vi "PicoLogHRDL2.vi"(1 "stop":bool, 2 "Mains Frequency":i16(ring) items=["50 Hz", "60 Hz"], 3 "sampleInterval_ms":i32=1000, 4 "1":bool=TRUE) -> (0 "Waveform Graph":dynamicdata(graph))   [LabVIEW 2014]
uses:
  Instance           1 22Saved   HRDL_streaming .vi
  Instance           3 22Saved   HRDL_streaming .vi
  Instance           2 22Saved   HRDL_streaming .vi
  Instance           6 22Saved   HRDL_streaming .vi
  Instance           5 22Saved   HRDL_streaming .vi
  Instance           4 22Saved   HRDL_streaming .vi
  Instance          10 22Saved   HRDL_streaming .vi
  Instance           9 22Saved   HRDL_streaming .vi
  Instance           8 22Saved   HRDL_streaming .vi
  Instance           7 22Saved   HRDL_streaming .vi
  Instance          15 22Saved   HRDL_streaming .vi
  Instance          14 22Saved   HRDL_streaming .vi
  Instance          13 22Saved   HRDL_streaming .vi
  Instance          12 22Saved   HRDL_streaming .vi
  Instance          11 22Saved   HRDL_streaming .vi
  Instance          21 22Saved   HRDL_streaming .vi
  Instance          20 22Saved   HRDL_streaming .vi
  Instance          19 22Saved   HRDL_streaming .vi
  Instance          18 22Saved   HRDL_streaming .vi
  Instance          17 22Saved   HRDL_streaming .vi
  Instance          16 22Saved   HRDL_streaming .vi
  Instance          28 22Saved   HRDL_streaming .vi
  Instance          27 22Saved   HRDL_streaming .vi
  Instance          26 22Saved   HRDL_streaming .vi
  Instance          25 22Saved   HRDL_streaming .vi
  Instance          24 22Saved   HRDL_streaming .vi
  Instance          23 22Saved   HRDL_streaming .vi
  Instance          22 22Saved   HRDL_streaming .vi
  Instance          36 22Saved   HRDL_streaming .vi
  Instance          35 22Saved   HRDL_streaming .vi
  Instance          34 22Saved   HRDL_streaming .vi
  Instance          33 22Saved   HRDL_streaming .vi
  Instance          32 22Saved   HRDL_streaming .vi
  Instance          31 22Saved   HRDL_streaming .vi
  Instance          30 22Saved   HRDL_streaming .vi
  Instance          29 22Saved   HRDL_streaming .vi
  Instance          45 22Saved   HRDL_streaming .vi
  Instance          44 22Saved   HRDL_streaming .vi
  Instance          43 22Saved   HRDL_streaming .vi
  Instance          42 22Saved   HRDL_streaming .vi
  Instance          41 22Saved   HRDL_streaming .vi
  Instance          40 22Saved   HRDL_streaming .vi
  Instance          39 22Saved   HRDL_streaming .vi
  Instance          38 22Saved   HRDL_streaming .vi
  Instance          37 22Saved   HRDL_streaming .vi
  Instance          55 22Saved   HRDL_streaming .vi
  Instance          54 22Saved   HRDL_streaming .vi
  Instance          53 22Saved   HRDL_streaming .vi
  Instance          52 22Saved   HRDL_streaming .vi
  Instance          51 22Saved   HRDL_streaming .vi
  Instance          50 22Saved   HRDL_streaming .vi
  Instance          49 22Saved   HRDL_streaming .vi
  Instance          48 22Saved   HRDL_streaming .vi
  Instance          47 22Saved   HRDL_streaming .vi
  Instance          46 22Saved   HRDL_streaming .vi
  Instance          66 22Saved   HRDL_streaming .vi
  Instance          65 22Saved   HRDL_streaming .vi
  Instance          64 22Saved   HRDL_streaming .vi
  Instance          63 22Saved   HRDL_streaming .vi
  Instance          62 22Saved   HRDL_streaming .vi
  Instance          61 22Saved   HRDL_streaming .vi
  Instance          60 22Saved   HRDL_streaming .vi
  Instance          59 22Saved   HRDL_streaming .vi
  Instance          58 22Saved   HRDL_streaming .vi
  Instance          57 22Saved   HRDL_streaming .vi
  Instance          56 22Saved   HRDL_streaming .vi
  Instance          78 22Saved   HRDL_streaming .vi
  Instance          77 22Saved   HRDL_streaming .vi
  Instance          76 22Saved   HRDL_streaming .vi
  Instance          75 22Saved   HRDL_streaming .vi
  Instance          74 22Saved   HRDL_streaming .vi
  Instance          73 22Saved   HRDL_streaming .vi
  Instance          72 22Saved   HRDL_streaming .vi
  Instance          71 22Saved   HRDL_streaming .vi
  Instance          70 22Saved   HRDL_streaming .vi
  Instance          69 22Saved   HRDL_streaming .vi
  Instance          68 22Saved   HRDL_streaming .vi
  Instance          67 22Saved   HRDL_streaming .vi
  Instance          91 22Saved   HRDL_streaming .vi
  Instance          90 22Saved   HRDL_streaming .vi
  Instance          89 22Saved   HRDL_streaming .vi
  Instance          88 22Saved   HRDL_streaming .vi
  Instance          87 22Saved   HRDL_streaming .vi
  Instance          86 22Saved   HRDL_streaming .vi
  Instance          85 22Saved   HRDL_streaming .vi
  Instance          84 22Saved   HRDL_streaming .vi
  Instance          83 22Saved   HRDL_streaming .vi
  Instance          82 22Saved   HRDL_streaming .vi
  Instance          81 22Saved   HRDL_streaming .vi
  Instance          80 22Saved   HRDL_streaming .vi
  Instance          79 22Saved   HRDL_streaming .vi
  Instance         105 22Saved   HRDL_streaming .vi
  Instance         104 22Saved   HRDL_streaming .vi
  Instance         103 22Saved   HRDL_streaming .vi
  Instance         102 22Saved   HRDL_streaming .vi
  Instance         101 22Saved   HRDL_streaming .vi
  Instance         100 22Saved   HRDL_streaming .vi
  Instance          99 22Saved   HRDL_streaming .vi
  Instance          98 22Saved   HRDL_streaming .vi
  Instance          97 22Saved   HRDL_streaming .vi
  Instance          96 22Saved   HRDL_streaming .vi
  Instance          95 22Saved   HRDL_streaming .vi
  Instance          94 22Saved   HRDL_streaming .vi
  Instance          93 22Saved   HRDL_streaming .vi
  Instance          92 22Saved   HRDL_streaming .vi
  Instance         120 22Saved   HRDL_streaming .vi
  Instance         119 22Saved   HRDL_streaming .vi
  Instance         118 22Saved   HRDL_streaming .vi
  Instance         117 22Saved   HRDL_streaming .vi
  Instance         116 22Saved   HRDL_streaming .vi
  Instance         115 22Saved   HRDL_streaming .vi
  Instance         114 22Saved   HRDL_streaming .vi
  Instance         113 22Saved   HRDL_streaming .vi
  Instance         112 22Saved   HRDL_streaming .vi
  Instance         111 22Saved   HRDL_streaming .vi
  Instance         110 22Saved   HRDL_streaming .vi
  Instance         109 22Saved   HRDL_streaming .vi
  Instance         108 22Saved   HRDL_streaming .vi
  Instance         107 22Saved   HRDL_streaming .vi
  Instance         106 22Saved   HRDL_streaming .vi
  Instance         136 22Saved   HRDL_streaming .vi
  Instance         135 22Saved   HRDL_streaming .vi
  Instance         134 22Saved   HRDL_streaming .vi
  Instance         133 22Saved   HRDL_streaming .vi
  Instance         132 22Saved   HRDL_streaming .vi
  Instance         131 22Saved   HRDL_streaming .vi
  Instance         130 22Saved   HRDL_streaming .vi
  Instance         129 22Saved   HRDL_streaming .vi
  Instance         128 22Saved   HRDL_streaming .vi
  Instance         127 22Saved   HRDL_streaming .vi
  Instance         126 22Saved   HRDL_streaming .vi
  Instance         125 22Saved   HRDL_streaming .vi
  Instance         124 22Saved   HRDL_streaming .vi
  Instance         123 22Saved   HRDL_streaming .vi
  Instance         122 22Saved   HRDL_streaming .vi
  Instance         121 22Saved   HRDL_streaming .vi
  Instance         137 22Saved   HRDL_streaming .vi
  Instance         138 22Saved   HRDL_streaming .vi
  picohrdl.dll
panel:
  out "Unit Info":T1
  in  "conversionTime":i16(ring) items=["60 ms", "100 ms", "180 ms", "340 ms", "660 ms"]
  out "noOfChannels":i16=2
  in  "16":bool
  in  "15":bool
  in  "14":bool
  in  "13":bool
  in  "12":bool
  in  "11":bool
  in  "10":bool
  in  "9":bool
  in  "8":bool
  in  "7":bool
  in  "6":bool
  in  "5":bool
  in  "4":bool
  in  "3":bool
  in  "2":bool=TRUE
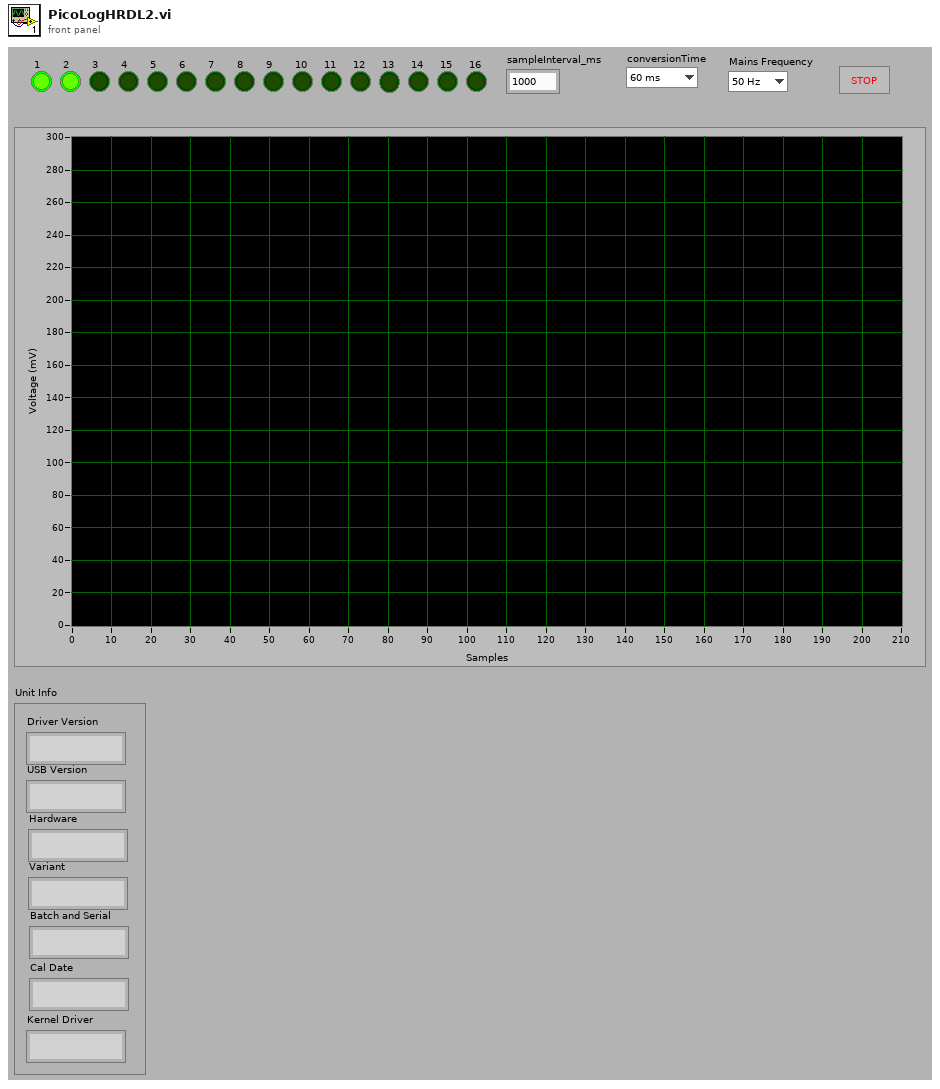
[diagram p1: front panel]
types:
  T1 = cluster{"Driver Version":string, "USB Version":string, "Hardware":string, "Variant":string, "Batch and Serial":string, "Cal Date":string, "Kernel Driver":string}
  T2 = cluster{"[0]":string, "[1]":string, "[2]":string, "[3]":string, "[4]":string, "[5]":string, "[6]":string}
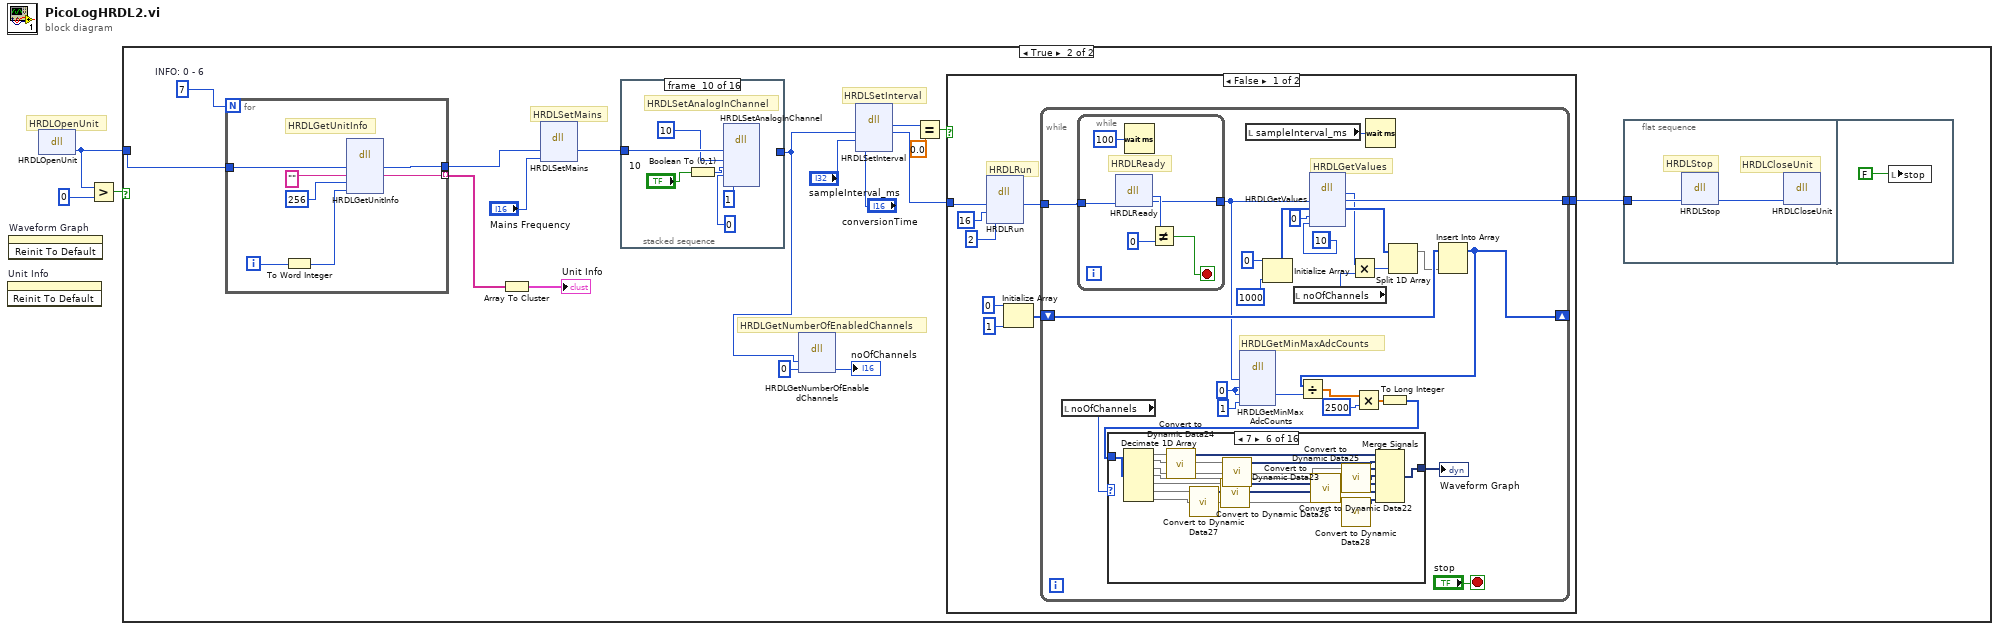
[diagram p0: block diagram]
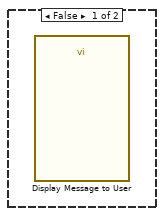
[diagram p2: hidden frame]
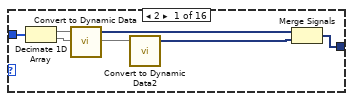
[diagram p3: hidden frame]
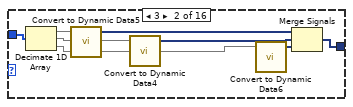
[diagram p4: hidden frame]
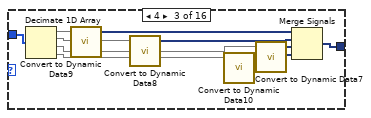
[diagram p5: hidden frame]
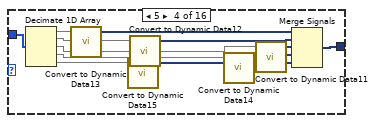
[diagram p6: hidden frame]
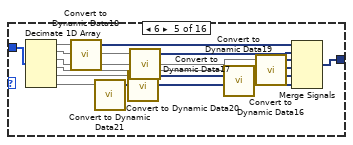
[diagram p7: hidden frame]
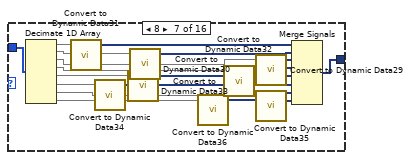
[diagram p8: hidden frame]
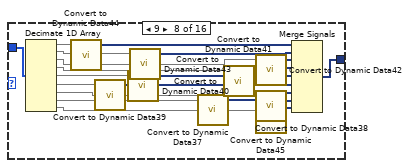
[diagram p9: hidden frame]
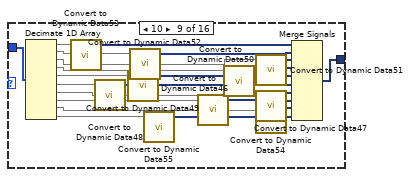
[diagram p10: hidden frame]
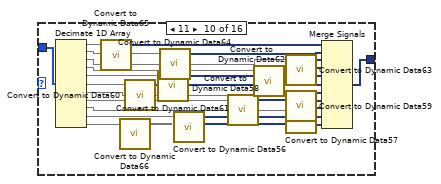
[diagram p11: hidden frame]
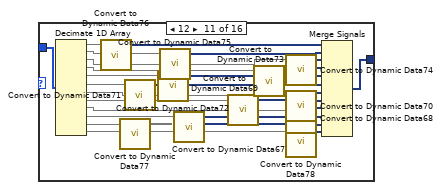
[diagram p12: hidden frame]
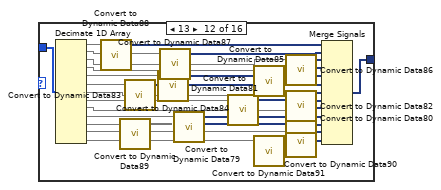
[diagram p13: hidden frame]
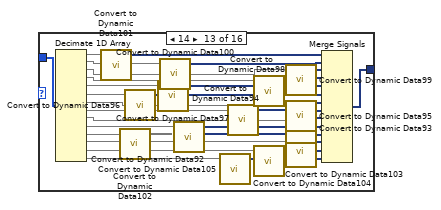
[diagram p14: hidden frame]
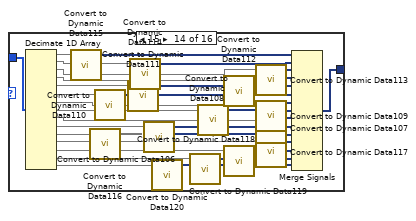
[diagram p15: hidden frame]
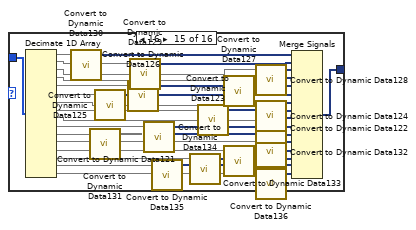
[diagram p16: hidden frame]
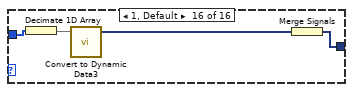
[diagram p17: hidden frame]
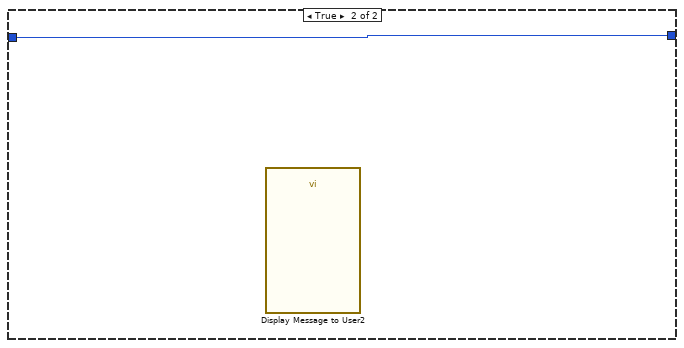
[diagram p18: hidden frame]
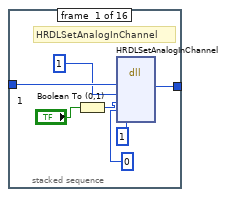
[diagram p19: hidden frame]
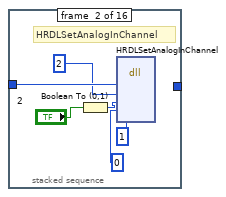
[diagram p20: hidden frame]
diagram:
  # "HRDLOpenUnit"
  n1 = invoke on="Unit Info" class="Clust (strict)" method="Reinit To Default"() -> ()  [unwired: 3 in, 3 out]
  n2 = invoke on="Waveform Graph" class="WFGraph (strict)" method="Reinit To Default"() -> ()  [unwired: 3 in, 3 out]
  n3 = dll-call lib="picohrdl.dll" fn="HRDLOpenUnit"() -> ("handle"=w1:i16)  [unwired: 3 in, 2 out]
  n4 = Greater?(x=w1, y=i16 0) -> (0:w3:bool)
  n5 = case shown="True" w3 {
    tunnel: w1 -> [_ w6]
    frame False {
      n6 = call "Display Message to User"() -> ()  [unwired: 10 in, 2 out]
    }
    frame True {
      w8 = 7  # INFO: 0 - 6
      # "HRDLGetNumberOfEnabledChannels"
      # "HRDLSetInterval"
      # "HRDLSetMains"
      n7 = for {
        N: w8 -> [_]
        tunnel: w6 -> [w27]
        tunnel: [w24] -> w5 mode=indexing
        tunnel: [w22] -> w7
        i -> [w23]
        # "HRDLGetUnitInfo"
        n8 = To Word Integer(number=w23) -> (16bit integer=w21:i16)
        n9 = dll-call lib="picohrdl.dll" fn="HRDLGetUnitInfo"("handle"=w27, "unitInfo"="", "stringLength"=i16 256, "info"=w21) -> ("handle"=w22:i16, "unitInfo"=w24:string)  [unwired: 6 in, 2 out]
      }
      n10 = Array To Cluster(array=w5) -> (cluster=→"Unit Info":T2)
      n11 = dll-call lib="PicoHRDL.dll" fn="HRDLSetMains"("handle"=w7, "sixtyHertz"="Mains Frequency") -> ("handle"=w11:i16)  [unwired: 5 in, 2 out]
      n12 = stacked-sequence {
        tunnel: w11 -> [w379 w385 w391 w397 w403 w409 w415 w421 w427 w433 w439 w445 w451 w457 w463 w469]
        tunnel: [w378 _ _ _ _ _ _ _ _ _ _ _ _ _ _ _] -> w9
        frame #0 {
          # "HRDLSetAnalogInChannel"
          n13 = Boolean To (0,1)(Boolean="1") -> (0, 1=w373:i16)
          n14 = dll-call lib="PicoHRDL.dll" fn="HRDLSetAnalogInChannel"("handle"=w379, "channel"=i16 1, "enabled"=w373, "range"=i16 0 ("range 1"), "singleEnded"=i16 1) -> ("handle"=w378:i16)  [unwired: 8 in, 2 out]
        }
        frame #1 {
          # "HRDLSetAnalogInChannel"
          n15 = Boolean To (0,1)(Boolean="2") -> (0, 1=w381:i16)
          n16 = dll-call lib="PicoHRDL.dll" fn="HRDLSetAnalogInChannel"("handle"=w385, "channel"=i16 2, "enabled"=w381, "range"=i16 0 ("range 2"), "singleEnded"=i16 1) -> ()  [unwired: 9 in, 2 out]
        }
        frame #2 {
          # "HRDLSetAnalogInChannel"
          n17 = Boolean To (0,1)(Boolean="3") -> (0, 1=w387:i16)
          n18 = dll-call lib="PicoHRDL.dll" fn="HRDLSetAnalogInChannel"("handle"=w391, "channel"=i16 3, "enabled"=w387, "range"=i16 0 ("range 3"), "singleEnded"=i16 1) -> ()  [unwired: 9 in, 2 out]
        }
        frame #3 {
          # "HRDLSetAnalogInChannel"
          n19 = Boolean To (0,1)(Boolean="4") -> (0, 1=w393:i16)
          n20 = dll-call lib="PicoHRDL.dll" fn="HRDLSetAnalogInChannel"("handle"=w397, "channel"=i16 4, "enabled"=w393, "range"=i16 0 ("range 4"), "singleEnded"=i16 1) -> ()  [unwired: 9 in, 2 out]
        }
        frame #4 {
          # "HRDLSetAnalogInChannel"
          n21 = Boolean To (0,1)(Boolean="5") -> (0, 1=w399:i16)
          n22 = dll-call lib="PicoHRDL.dll" fn="HRDLSetAnalogInChannel"("handle"=w403, "channel"=i16 5, "enabled"=w399, "range"=i16 0 ("range 5"), "singleEnded"=i16 1) -> ()  [unwired: 9 in, 2 out]
        }
        frame #5 {
          # "HRDLSetAnalogInChannel"
          n23 = Boolean To (0,1)(Boolean="6") -> (0, 1=w405:i16)
          n24 = dll-call lib="PicoHRDL.dll" fn="HRDLSetAnalogInChannel"("handle"=w409, "channel"=i16 6, "enabled"=w405, "range"=i16 0 ("range 6"), "singleEnded"=i16 1) -> ()  [unwired: 9 in, 2 out]
        }
        frame #6 {
          # "HRDLSetAnalogInChannel"
          n25 = Boolean To (0,1)(Boolean="7") -> (0, 1=w411:i16)
          n26 = dll-call lib="PicoHRDL.dll" fn="HRDLSetAnalogInChannel"("handle"=w415, "channel"=i16 7, "enabled"=w411, "range"=i16 0 ("range 7"), "singleEnded"=i16 1) -> ()  [unwired: 9 in, 2 out]
        }
        frame #7 {
          # "HRDLSetAnalogInChannel"
          n27 = Boolean To (0,1)(Boolean="8") -> (0, 1=w417:i16)
          n28 = dll-call lib="PicoHRDL.dll" fn="HRDLSetAnalogInChannel"("handle"=w421, "channel"=i16 8, "enabled"=w417, "range"=i16 0 ("range 8"), "singleEnded"=i16 1) -> ()  [unwired: 9 in, 2 out]
        }
        frame #8 {
          # "HRDLSetAnalogInChannel"
          n29 = Boolean To (0,1)(Boolean="9") -> (0, 1=w423:i16)
          n30 = dll-call lib="PicoHRDL.dll" fn="HRDLSetAnalogInChannel"("handle"=w427, "channel"=i16 9, "enabled"=w423, "range"=i16 0 ("range 9"), "singleEnded"=i16 1) -> ()  [unwired: 9 in, 2 out]
        }
        frame #9 {
          # "HRDLSetAnalogInChannel"
          n31 = Boolean To (0,1)(Boolean="10") -> (0, 1=w429:i16)
          n32 = dll-call lib="PicoHRDL.dll" fn="HRDLSetAnalogInChannel"("handle"=w433, "channel"=i16 10, "enabled"=w429, "range"=i16 0 ("range 10"), "singleEnded"=i16 1) -> ()  [unwired: 9 in, 2 out]
        }
        frame #10 {
          # "HRDLSetAnalogInChannel"
          n33 = Boolean To (0,1)(Boolean="11") -> (0, 1=w435:i16)
          n34 = dll-call lib="PicoHRDL.dll" fn="HRDLSetAnalogInChannel"("handle"=w439, "channel"=i16 11, "enabled"=w435, "range"=i16 0 ("range 11"), "singleEnded"=i16 1) -> ()  [unwired: 9 in, 2 out]
        }
        frame #11 {
          # "HRDLSetAnalogInChannel"
          n35 = Boolean To (0,1)(Boolean="12") -> (0, 1=w441:i16)
          n36 = dll-call lib="PicoHRDL.dll" fn="HRDLSetAnalogInChannel"("handle"=w445, "channel"=i16 12, "enabled"=w441, "range"=i16 0 ("range 12"), "singleEnded"=i16 1) -> ()  [unwired: 9 in, 2 out]
        }
        frame #12 {
          # "HRDLSetAnalogInChannel"
          n37 = Boolean To (0,1)(Boolean="13") -> (0, 1=w447:i16)
          n38 = dll-call lib="PicoHRDL.dll" fn="HRDLSetAnalogInChannel"("handle"=w451, "channel"=i16 13, "enabled"=w447, "range"=i16 0 ("range 13"), "singleEnded"=i16 1) -> ()  [unwired: 9 in, 2 out]
        }
        frame #13 {
          # "HRDLSetAnalogInChannel"
          n39 = Boolean To (0,1)(Boolean="14") -> (0, 1=w453:i16)
          n40 = dll-call lib="PicoHRDL.dll" fn="HRDLSetAnalogInChannel"("handle"=w457, "channel"=i16 14, "enabled"=w453, "range"=i16 0 ("range 14"), "singleEnded"=i16 1) -> ()  [unwired: 9 in, 2 out]
        }
        frame #14 {
          # "HRDLSetAnalogInChannel"
          n41 = Boolean To (0,1)(Boolean="15") -> (0, 1=w459:i16)
          n42 = dll-call lib="PicoHRDL.dll" fn="HRDLSetAnalogInChannel"("handle"=w463, "channel"=i16 15, "enabled"=w459, "range"=i16 0 ("range 15"), "singleEnded"=i16 1) -> ()  [unwired: 9 in, 2 out]
        }
        frame #15 {
          # "HRDLSetAnalogInChannel"
          n43 = Boolean To (0,1)(Boolean="16") -> (0, 1=w465:i16)
          n44 = dll-call lib="PicoHRDL.dll" fn="HRDLSetAnalogInChannel"("handle"=w469, "channel"=i16 16, "enabled"=w465, "range"=i16 0 ("range 16"), "singleEnded"=i16 1) -> ()  [unwired: 9 in, 2 out]
        }
      }
      n45 = dll-call lib="PicoHRDL.dll" fn="HRDLGetNumberOfEnabledChannels"("handle"=w9, "nEnabledChannels"=i16 0) -> ("nEnabledChannels"=→"noOfChannels":i16)  [unwired: 5 in, 2 out]
      n46 = dll-call lib="PicoHRDL.dll" fn="HRDLSetInterval"("handle"=w9, "sampleInterval_ms"="sampleInterval_ms", "conversionTime"="conversionTime") -> ("return type"=w15:i16, "handle"=w14:i16)  [unwired: 5 in, 2 out]
      n47 = Equal?(x=w15, y=0.0) -> (x = y?=w13:bool)
      n48 = case shown="False" w13 {
        tunnel: [w32 w372] -> w20
        tunnel: w14 -> [w28 w372]
        frame False {
          # "HRDLRun"
          n49 = dll-call lib="PicoHRDL.dll" fn="HRDLRun"("handle"=w28, "nValues"=16, "method"=i16 2) -> ("handle"=w33:i16)  [unwired: 6 in, 2 out]
          n50 = Initialize Array(0 ("element"), 1 ("dimension size")) -> (w29:i32[])
          n51 = while {
            tunnel: w33 -> [w61]
            tunnel: [w55] -> w32
            shift-right: [w48] -> _
            shift-left: w29 -> [w49]
            stop <- "stop" stop-if-true
            w53 = 0 ("maxAdc")
            (unwired) 10 ("noOfValues")
            # "HRDLGetMinMaxAdcCounts"
            # "HRDLGetValues"
            n52 = local read "noOfChannels"() -> (w42:i16)
            n53 = while {
              tunnel: w61 -> [w368]
              tunnel: [w367] -> w38
              stop <- w369 stop-if-true
              # "HRDLReady"
              n54 = dll-call lib="PicoHRDL.dll" fn="HRDLReady"("handle"=w368) -> ("ready"=w371:i16, "handle"=w367:i16)  [unwired: 3 in, 2 out]
              n55 = Wait (ms)(milliseconds to wait=u32 100) -> ()  [unwired: 1 out]
              n56 = Not Equal?(x=w371, y=i16 0) -> (x != y?=w369:bool)
            }
            n57 = dll-call lib="PicoHRDL.dll" fn="HRDLGetMinMaxAdcCounts"("handle"=w38, "minAdc"=w53, "maxAdc"=w53, "channel"=i16 1) -> ("maxAdc"=w39:i32)  [unwired: 7 in, 2 out]
            n58 = local read "sampleInterval_ms"() -> (w36:i32)
            n59 = Initialize Array(0 ("element"), 1000 ("dimension size")) -> (w60:i32[])
            n60 = local read "noOfChannels"() -> (w46:i16)
            n61 = dll-call lib="PicoHRDL.dll" fn="HRDLGetValues"("handle"=w38, "values"=w60, "overflow"=i16 0, "noOfValues"=10) -> ("noValuesPerChan"=w44:i32, "handle"=w55:i16, "values"=w47:i32[])  [unwired: 5 in, 2 out]
            n62 = Multiply(x=w44, y=w46) -> (x*y=w45:i32)
            n63 = Wait (ms)(milliseconds to wait=w36) -> ()  [unwired: 1 out]
            n64 = Split 1D Array(array=w47, index=w45) -> (first subarray=w43:i32[])  [unwired: 1 out]
            n65 = Insert Into Array(array=w49, new element=w43) -> (w48:i32[])  [unwired: 1 in]
            n66 = Divide(x=w48, y=w39) -> (x/y=w52:dbl[])
            n67 = Multiply(x=w52, y=2500 ("noOfValues")) -> (x*y=w51:dbl[])
            n68 = To Long Integer(number=w51) -> (32bit integer=w40:i32[])
            n69 = case shown="7" w42 {
              tunnel: [w63 w71 w81 w93 w107 w123 w141 w161 w183 w207 w233 w261 w291 w323 w357 w363] -> w41
              tunnel: w40 -> [w62 w70 w80 w92 w106 w122 w140 w160 w182 w206 w232 w260 w290 w322 w356 w362]
              frame 2 {
                n70 = Decimate 1D Array(w62) -> (w64:i32[], w66:i32[])
                n71 = call "Convert to Dynamic Data"("Array"=w64) -> ("Dynamic Data Type"=w65:dynamicdata)  [unwired: 3 in]
                n72 = call "Convert to Dynamic Data2"("Array"=w66) -> ("Dynamic Data Type"=w67:dynamicdata)  [unwired: 3 in]
                n73 = Merge Signals(w65, w67) -> (w63:dynamicdata)
              }
              frame 3 {
                n74 = Decimate 1D Array(w70) -> (w72:i32[], w74:i32[], w69:i32[])
                n75 = call "Convert to Dynamic Data5"("Array"=w72) -> ("Dynamic Data Type"=w73:dynamicdata)  [unwired: 3 in]
                n76 = call "Convert to Dynamic Data4"("Array"=w74) -> ("Dynamic Data Type"=w75:dynamicdata)  [unwired: 3 in]
                n77 = call "Convert to Dynamic Data6"("Array"=w69) -> ("Dynamic Data Type"=w68:dynamicdata)  [unwired: 3 in]
                n78 = Merge Signals(w73, w75, w68) -> (w71:dynamicdata)
              }
              frame 4 {
                n79 = Decimate 1D Array(w80) -> (w82:i32[], w84:i32[], w79:i32[], w77:i32[])
                n80 = call "Convert to Dynamic Data9"("Array"=w82) -> ("Dynamic Data Type"=w83:dynamicdata)  [unwired: 3 in]
                n81 = call "Convert to Dynamic Data8"("Array"=w84) -> ("Dynamic Data Type"=w85:dynamicdata)  [unwired: 3 in]
                n82 = call "Convert to Dynamic Data10"("Array"=w77) -> ("Dynamic Data Type"=w76:dynamicdata)  [unwired: 3 in]
                n83 = call "Convert to Dynamic Data7"("Array"=w79) -> ("Dynamic Data Type"=w78:dynamicdata)  [unwired: 3 in]
                n84 = Merge Signals(w83, w85, w78, w76) -> (w81:dynamicdata)
              }
              frame 5 {
                n85 = Decimate 1D Array(w92) -> (w94:i32[], w96:i32[], w91:i32[], w89:i32[], w87:i32[])
                n86 = call "Convert to Dynamic Data13"("Array"=w94) -> ("Dynamic Data Type"=w95:dynamicdata)  [unwired: 3 in]
                n87 = call "Convert to Dynamic Data15"("Array"=w87) -> ("Dynamic Data Type"=w86:dynamicdata)  [unwired: 3 in]
                n88 = call "Convert to Dynamic Data12"("Array"=w96) -> ("Dynamic Data Type"=w97:dynamicdata)  [unwired: 3 in]
                n89 = call "Convert to Dynamic Data14"("Array"=w89) -> ("Dynamic Data Type"=w88:dynamicdata)  [unwired: 3 in]
                n90 = call "Convert to Dynamic Data11"("Array"=w91) -> ("Dynamic Data Type"=w90:dynamicdata)  [unwired: 3 in]
                n91 = Merge Signals(w95, w97, w90, w88, w86) -> (w93:dynamicdata)
              }
              frame 6 {
                n92 = Decimate 1D Array(w106) -> (w108:i32[], w110:i32[], w105:i32[], w103:i32[], w101:i32[], w99:i32[])
                n93 = call "Convert to Dynamic Data18"("Array"=w108) -> ("Dynamic Data Type"=w109:dynamicdata)  [unwired: 3 in]
                n94 = call "Convert to Dynamic Data21"("Array"=w99) -> ("Dynamic Data Type"=w98:dynamicdata)  [unwired: 3 in]
                n95 = call "Convert to Dynamic Data20"("Array"=w101) -> ("Dynamic Data Type"=w100:dynamicdata)  [unwired: 3 in]
                n96 = call "Convert to Dynamic Data17"("Array"=w110) -> ("Dynamic Data Type"=w111:dynamicdata)  [unwired: 3 in]
                n97 = call "Convert to Dynamic Data19"("Array"=w103) -> ("Dynamic Data Type"=w102:dynamicdata)  [unwired: 3 in]
                n98 = call "Convert to Dynamic Data16"("Array"=w105) -> ("Dynamic Data Type"=w104:dynamicdata)  [unwired: 3 in]
                n99 = Merge Signals(w109, w111, w104, w102, w100, w98) -> (w107:dynamicdata)
              }
              frame 7 {
                n100 = Decimate 1D Array(w122) -> (w124:i32[], w126:i32[], w121:i32[], w119:i32[], w117:i32[], w115:i32[], w113:i32[])
                n101 = call "Convert to Dynamic Data24"("Array"=w124) -> ("Dynamic Data Type"=w125:dynamicdata)  [unwired: 3 in]
                n102 = call "Convert to Dynamic Data27"("Array"=w115) -> ("Dynamic Data Type"=w114:dynamicdata)  [unwired: 3 in]
                n103 = call "Convert to Dynamic Data26"("Array"=w117) -> ("Dynamic Data Type"=w116:dynamicdata)  [unwired: 3 in]
                n104 = call "Convert to Dynamic Data23"("Array"=w126) -> ("Dynamic Data Type"=w127:dynamicdata)  [unwired: 3 in]
                n105 = call "Convert to Dynamic Data25"("Array"=w119) -> ("Dynamic Data Type"=w118:dynamicdata)  [unwired: 3 in]
                n106 = call "Convert to Dynamic Data22"("Array"=w121) -> ("Dynamic Data Type"=w120:dynamicdata)  [unwired: 3 in]
                n107 = call "Convert to Dynamic Data28"("Array"=w113) -> ("Dynamic Data Type"=w112:dynamicdata)  [unwired: 3 in]
                n108 = Merge Signals(w125, w127, w120, w118, w116, w114, w112) -> (w123:dynamicdata)
              }
              frame 8 {
                n109 = Decimate 1D Array(w140) -> (w142:i32[], w144:i32[], w139:i32[], w137:i32[], w135:i32[], w133:i32[], w131:i32[], w129:i32[])
                n110 = call "Convert to Dynamic Data31"("Array"=w142) -> ("Dynamic Data Type"=w143:dynamicdata)  [unwired: 3 in]
                n111 = call "Convert to Dynamic Data34"("Array"=w133) -> ("Dynamic Data Type"=w132:dynamicdata)  [unwired: 3 in]
                n112 = call "Convert to Dynamic Data33"("Array"=w135) -> ("Dynamic Data Type"=w134:dynamicdata)  [unwired: 3 in]
                n113 = call "Convert to Dynamic Data30"("Array"=w144) -> ("Dynamic Data Type"=w145:dynamicdata)  [unwired: 3 in]
                n114 = call "Convert to Dynamic Data36"("Array"=w129) -> ("Dynamic Data Type"=w128:dynamicdata)  [unwired: 3 in]
                n115 = call "Convert to Dynamic Data32"("Array"=w137) -> ("Dynamic Data Type"=w136:dynamicdata)  [unwired: 3 in]
                n116 = call "Convert to Dynamic Data29"("Array"=w139) -> ("Dynamic Data Type"=w138:dynamicdata)  [unwired: 3 in]
                n117 = call "Convert to Dynamic Data35"("Array"=w131) -> ("Dynamic Data Type"=w130:dynamicdata)  [unwired: 3 in]
                n118 = Merge Signals(w143, w145, w138, w136, w134, w132, w130, w128) -> (w141:dynamicdata)
              }
              frame 9 {
                n119 = Decimate 1D Array(w160) -> (w162:i32[], w164:i32[], w159:i32[], w157:i32[], w155:i32[], w153:i32[], w151:i32[], w149:i32[], w147:i32[])
                n120 = call "Convert to Dynamic Data44"("Array"=w162) -> ("Dynamic Data Type"=w163:dynamicdata)  [unwired: 3 in]
                n121 = call "Convert to Dynamic Data39"("Array"=w153) -> ("Dynamic Data Type"=w152:dynamicdata)  [unwired: 3 in]
                n122 = call "Convert to Dynamic Data40"("Array"=w155) -> ("Dynamic Data Type"=w154:dynamicdata)  [unwired: 3 in]
                n123 = call "Convert to Dynamic Data43"("Array"=w164) -> ("Dynamic Data Type"=w165:dynamicdata)  [unwired: 3 in]
                n124 = call "Convert to Dynamic Data37"("Array"=w149) -> ("Dynamic Data Type"=w148:dynamicdata)  [unwired: 3 in]
                n125 = call "Convert to Dynamic Data41"("Array"=w157) -> ("Dynamic Data Type"=w156:dynamicdata)  [unwired: 3 in]
                n126 = call "Convert to Dynamic Data42"("Array"=w159) -> ("Dynamic Data Type"=w158:dynamicdata)  [unwired: 3 in]
                n127 = call "Convert to Dynamic Data38"("Array"=w151) -> ("Dynamic Data Type"=w150:dynamicdata)  [unwired: 3 in]
                n128 = call "Convert to Dynamic Data45"("Array"=w147) -> ("Dynamic Data Type"=w146:dynamicdata)  [unwired: 3 in]
                n129 = Merge Signals(w163, w165, w158, w156, w154, w152, w150, w148, w146) -> (w161:dynamicdata)
              }
              frame 10 {
                n130 = Decimate 1D Array(w182) -> (w184:i32[], w186:i32[], w181:i32[], w179:i32[], w177:i32[], w175:i32[], w173:i32[], w171:i32[], w169:i32[], w167:i32[])
                n131 = call "Convert to Dynamic Data53"("Array"=w184) -> ("Dynamic Data Type"=w185:dynamicdata)  [unwired: 3 in]
                n132 = call "Convert to Dynamic Data48"("Array"=w175) -> ("Dynamic Data Type"=w174:dynamicdata)  [unwired: 3 in]
                n133 = call "Convert to Dynamic Data49"("Array"=w177) -> ("Dynamic Data Type"=w176:dynamicdata)  [unwired: 3 in]
                n134 = call "Convert to Dynamic Data52"("Array"=w186) -> ("Dynamic Data Type"=w187:dynamicdata)  [unwired: 3 in]
                n135 = call "Convert to Dynamic Data55"("Array"=w167) -> ("Dynamic Data Type"=w166:dynamicdata)  [unwired: 3 in]
                n136 = call "Convert to Dynamic Data46"("Array"=w171) -> ("Dynamic Data Type"=w170:dynamicdata)  [unwired: 3 in]
                n137 = call "Convert to Dynamic Data50"("Array"=w179) -> ("Dynamic Data Type"=w178:dynamicdata)  [unwired: 3 in]
                n138 = call "Convert to Dynamic Data51"("Array"=w181) -> ("Dynamic Data Type"=w180:dynamicdata)  [unwired: 3 in]
                n139 = call "Convert to Dynamic Data47"("Array"=w173) -> ("Dynamic Data Type"=w172:dynamicdata)  [unwired: 3 in]
                n140 = call "Convert to Dynamic Data54"("Array"=w169) -> ("Dynamic Data Type"=w168:dynamicdata)  [unwired: 3 in]
                n141 = Merge Signals(w185, w187, w180, w178, w176, w174, w172, w170, w168, w166) -> (w183:dynamicdata)
              }
              frame 11 {
                n142 = Decimate 1D Array(w206) -> (w208:i32[], w210:i32[], w205:i32[], w203:i32[], w201:i32[], w199:i32[], w197:i32[], w195:i32[], w193:i32[], w191:i32[], w189:i32[])
                n143 = call "Convert to Dynamic Data65"("Array"=w208) -> ("Dynamic Data Type"=w209:dynamicdata)  [unwired: 3 in]
                n144 = call "Convert to Dynamic Data66"("Array"=w189) -> ("Dynamic Data Type"=w188:dynamicdata)  [unwired: 3 in]
                n145 = call "Convert to Dynamic Data60"("Array"=w199) -> ("Dynamic Data Type"=w198:dynamicdata)  [unwired: 3 in]
                n146 = call "Convert to Dynamic Data61"("Array"=w201) -> ("Dynamic Data Type"=w200:dynamicdata)  [unwired: 3 in]
                n147 = call "Convert to Dynamic Data64"("Array"=w210) -> ("Dynamic Data Type"=w211:dynamicdata)  [unwired: 3 in]
                n148 = call "Convert to Dynamic Data56"("Array"=w191) -> ("Dynamic Data Type"=w190:dynamicdata)  [unwired: 3 in]
                n149 = call "Convert to Dynamic Data58"("Array"=w195) -> ("Dynamic Data Type"=w194:dynamicdata)  [unwired: 3 in]
                n150 = call "Convert to Dynamic Data62"("Array"=w203) -> ("Dynamic Data Type"=w202:dynamicdata)  [unwired: 3 in]
                n151 = call "Convert to Dynamic Data63"("Array"=w205) -> ("Dynamic Data Type"=w204:dynamicdata)  [unwired: 3 in]
                n152 = call "Convert to Dynamic Data59"("Array"=w197) -> ("Dynamic Data Type"=w196:dynamicdata)  [unwired: 3 in]
                n153 = call "Convert to Dynamic Data57"("Array"=w193) -> ("Dynamic Data Type"=w192:dynamicdata)  [unwired: 3 in]
                n154 = Merge Signals(w209, w211, w204, w202, w200, w198, w196, w194, w192, w190, w188) -> (w207:dynamicdata)
              }
              frame 12 {
                n155 = Decimate 1D Array(w232) -> (w234:i32[], w236:i32[], w231:i32[], w229:i32[], w227:i32[], w225:i32[], w223:i32[], w221:i32[], w219:i32[], w217:i32[], w215:i32[], w213:i32[])
                n156 = call "Convert to Dynamic Data76"("Array"=w234) -> ("Dynamic Data Type"=w235:dynamicdata)  [unwired: 3 in]
                n157 = call "Convert to Dynamic Data77"("Array"=w215) -> ("Dynamic Data Type"=w214:dynamicdata)  [unwired: 3 in]
                n158 = call "Convert to Dynamic Data71"("Array"=w225) -> ("Dynamic Data Type"=w224:dynamicdata)  [unwired: 3 in]
                n159 = call "Convert to Dynamic Data72"("Array"=w227) -> ("Dynamic Data Type"=w226:dynamicdata)  [unwired: 3 in]
                n160 = call "Convert to Dynamic Data75"("Array"=w236) -> ("Dynamic Data Type"=w237:dynamicdata)  [unwired: 3 in]
                n161 = call "Convert to Dynamic Data67"("Array"=w217) -> ("Dynamic Data Type"=w216:dynamicdata)  [unwired: 3 in]
                n162 = call "Convert to Dynamic Data69"("Array"=w221) -> ("Dynamic Data Type"=w220:dynamicdata)  [unwired: 3 in]
                n163 = call "Convert to Dynamic Data73"("Array"=w229) -> ("Dynamic Data Type"=w228:dynamicdata)  [unwired: 3 in]
                n164 = call "Convert to Dynamic Data74"("Array"=w231) -> ("Dynamic Data Type"=w230:dynamicdata)  [unwired: 3 in]
                n165 = call "Convert to Dynamic Data70"("Array"=w223) -> ("Dynamic Data Type"=w222:dynamicdata)  [unwired: 3 in]
                n166 = call "Convert to Dynamic Data68"("Array"=w219) -> ("Dynamic Data Type"=w218:dynamicdata)  [unwired: 3 in]
                n167 = call "Convert to Dynamic Data78"("Array"=w213) -> ("Dynamic Data Type"=w212:dynamicdata)  [unwired: 3 in]
                n168 = Merge Signals(w235, w237, w230, w228, w226, w224, w222, w220, w218, w216, w214, w212) -> (w233:dynamicdata)
              }
              frame 13 {
                n169 = Decimate 1D Array(w260) -> (w262:i32[], w264:i32[], w259:i32[], w257:i32[], w255:i32[], w253:i32[], w251:i32[], w249:i32[], w247:i32[], w245:i32[], w243:i32[], w241:i32[], w239:i32[])
                n170 = call "Convert to Dynamic Data88"("Array"=w262) -> ("Dynamic Data Type"=w263:dynamicdata)  [unwired: 3 in]
                n171 = call "Convert to Dynamic Data89"("Array"=w243) -> ("Dynamic Data Type"=w242:dynamicdata)  [unwired: 3 in]
                n172 = call "Convert to Dynamic Data83"("Array"=w253) -> ("Dynamic Data Type"=w252:dynamicdata)  [unwired: 3 in]
                n173 = call "Convert to Dynamic Data84"("Array"=w255) -> ("Dynamic Data Type"=w254:dynamicdata)  [unwired: 3 in]
                n174 = call "Convert to Dynamic Data87"("Array"=w264) -> ("Dynamic Data Type"=w265:dynamicdata)  [unwired: 3 in]
                n175 = call "Convert to Dynamic Data79"("Array"=w245) -> ("Dynamic Data Type"=w244:dynamicdata)  [unwired: 3 in]
                n176 = call "Convert to Dynamic Data81"("Array"=w249) -> ("Dynamic Data Type"=w248:dynamicdata)  [unwired: 3 in]
                n177 = call "Convert to Dynamic Data85"("Array"=w257) -> ("Dynamic Data Type"=w256:dynamicdata)  [unwired: 3 in]
                n178 = call "Convert to Dynamic Data91"("Array"=w239) -> ("Dynamic Data Type"=w238:dynamicdata)  [unwired: 3 in]
                n179 = call "Convert to Dynamic Data86"("Array"=w259) -> ("Dynamic Data Type"=w258:dynamicdata)  [unwired: 3 in]
                n180 = call "Convert to Dynamic Data82"("Array"=w251) -> ("Dynamic Data Type"=w250:dynamicdata)  [unwired: 3 in]
                n181 = call "Convert to Dynamic Data80"("Array"=w247) -> ("Dynamic Data Type"=w246:dynamicdata)  [unwired: 3 in]
                n182 = call "Convert to Dynamic Data90"("Array"=w241) -> ("Dynamic Data Type"=w240:dynamicdata)  [unwired: 3 in]
                n183 = Merge Signals(w263, w265, w258, w256, w254, w252, w250, w248, w246, w244, w242, w240, w238) -> (w261:dynamicdata)
              }
              frame 14 {
                n184 = Decimate 1D Array(w290) -> (w292:i32[], w294:i32[], w289:i32[], w287:i32[], w285:i32[], w283:i32[], w281:i32[], w279:i32[], w277:i32[], w275:i32[], w273:i32[], w271:i32[], w269:i32[], w267:i32[])
                n185 = call "Convert to Dynamic Data101"("Array"=w292) -> ("Dynamic Data Type"=w293:dynamicdata)  [unwired: 3 in]
                n186 = call "Convert to Dynamic Data102"("Array"=w273) -> ("Dynamic Data Type"=w272:dynamicdata)  [unwired: 3 in]
                n187 = call "Convert to Dynamic Data96"("Array"=w283) -> ("Dynamic Data Type"=w282:dynamicdata)  [unwired: 3 in]
                n188 = call "Convert to Dynamic Data97"("Array"=w285) -> ("Dynamic Data Type"=w284:dynamicdata)  [unwired: 3 in]
                n189 = call "Convert to Dynamic Data100"("Array"=w294) -> ("Dynamic Data Type"=w295:dynamicdata)  [unwired: 3 in]
                n190 = call "Convert to Dynamic Data92"("Array"=w275) -> ("Dynamic Data Type"=w274:dynamicdata)  [unwired: 3 in]
                n191 = call "Convert to Dynamic Data105"("Array"=w267) -> ("Dynamic Data Type"=w266:dynamicdata)  [unwired: 3 in]
                n192 = call "Convert to Dynamic Data94"("Array"=w279) -> ("Dynamic Data Type"=w278:dynamicdata)  [unwired: 3 in]
                n193 = call "Convert to Dynamic Data98"("Array"=w287) -> ("Dynamic Data Type"=w286:dynamicdata)  [unwired: 3 in]
                n194 = call "Convert to Dynamic Data104"("Array"=w269) -> ("Dynamic Data Type"=w268:dynamicdata)  [unwired: 3 in]
                n195 = call "Convert to Dynamic Data99"("Array"=w289) -> ("Dynamic Data Type"=w288:dynamicdata)  [unwired: 3 in]
                n196 = call "Convert to Dynamic Data95"("Array"=w281) -> ("Dynamic Data Type"=w280:dynamicdata)  [unwired: 3 in]
                n197 = call "Convert to Dynamic Data93"("Array"=w277) -> ("Dynamic Data Type"=w276:dynamicdata)  [unwired: 3 in]
                n198 = call "Convert to Dynamic Data103"("Array"=w271) -> ("Dynamic Data Type"=w270:dynamicdata)  [unwired: 3 in]
                n199 = Merge Signals(w293, w295, w288, w286, w284, w282, w280, w278, w276, w274, w272, w270, w268, w266) -> (w291:dynamicdata)
              }
              frame 15 {
                n200 = Decimate 1D Array(w322) -> (w324:i32[], w326:i32[], w321:i32[], w319:i32[], w317:i32[], w315:i32[], w313:i32[], w311:i32[], w309:i32[], w307:i32[], w305:i32[], w303:i32[], w301:i32[], w299:i32[], w297:i32[])
                n201 = call "Convert to Dynamic Data115"("Array"=w324) -> ("Dynamic Data Type"=w325:dynamicdata)  [unwired: 3 in]
                n202 = call "Convert to Dynamic Data116"("Array"=w305) -> ("Dynamic Data Type"=w304:dynamicdata)  [unwired: 3 in]
                n203 = call "Convert to Dynamic Data110"("Array"=w315) -> ("Dynamic Data Type"=w314:dynamicdata)  [unwired: 3 in]
                n204 = call "Convert to Dynamic Data111"("Array"=w317) -> ("Dynamic Data Type"=w316:dynamicdata)  [unwired: 3 in]
                n205 = call "Convert to Dynamic Data114"("Array"=w326) -> ("Dynamic Data Type"=w327:dynamicdata)  [unwired: 3 in]
                n206 = call "Convert to Dynamic Data106"("Array"=w307) -> ("Dynamic Data Type"=w306:dynamicdata)  [unwired: 3 in]
                n207 = call "Convert to Dynamic Data120"("Array"=w297) -> ("Dynamic Data Type"=w296:dynamicdata)  [unwired: 3 in]
                n208 = call "Convert to Dynamic Data119"("Array"=w299) -> ("Dynamic Data Type"=w298:dynamicdata)  [unwired: 3 in]
                n209 = call "Convert to Dynamic Data108"("Array"=w311) -> ("Dynamic Data Type"=w310:dynamicdata)  [unwired: 3 in]
                n210 = call "Convert to Dynamic Data112"("Array"=w319) -> ("Dynamic Data Type"=w318:dynamicdata)  [unwired: 3 in]
                n211 = call "Convert to Dynamic Data118"("Array"=w301) -> ("Dynamic Data Type"=w300:dynamicdata)  [unwired: 3 in]
                n212 = call "Convert to Dynamic Data113"("Array"=w321) -> ("Dynamic Data Type"=w320:dynamicdata)  [unwired: 3 in]
                n213 = call "Convert to Dynamic Data109"("Array"=w313) -> ("Dynamic Data Type"=w312:dynamicdata)  [unwired: 3 in]
                n214 = call "Convert to Dynamic Data107"("Array"=w309) -> ("Dynamic Data Type"=w308:dynamicdata)  [unwired: 3 in]
                n215 = call "Convert to Dynamic Data117"("Array"=w303) -> ("Dynamic Data Type"=w302:dynamicdata)  [unwired: 3 in]
                n216 = Merge Signals(w325, w327, w320, w318, w316, w314, w312, w310, w308, w306, w304, w302, w300, w298, w296) -> (w323:dynamicdata)
              }
              frame 16 {
                n217 = Decimate 1D Array(w356) -> (w358:i32[], w360:i32[], w355:i32[], w353:i32[], w351:i32[], w349:i32[], w347:i32[], w345:i32[], w343:i32[], w341:i32[], w339:i32[], w337:i32[], w335:i32[], w333:i32[], w331:i32[], w329:i32[])
                n218 = call "Convert to Dynamic Data130"("Array"=w358) -> ("Dynamic Data Type"=w359:dynamicdata)  [unwired: 3 in]
                n219 = call "Convert to Dynamic Data131"("Array"=w339) -> ("Dynamic Data Type"=w338:dynamicdata)  [unwired: 3 in]
                n220 = call "Convert to Dynamic Data125"("Array"=w349) -> ("Dynamic Data Type"=w348:dynamicdata)  [unwired: 3 in]
                n221 = call "Convert to Dynamic Data126"("Array"=w351) -> ("Dynamic Data Type"=w350:dynamicdata)  [unwired: 3 in]
                n222 = call "Convert to Dynamic Data129"("Array"=w360) -> ("Dynamic Data Type"=w361:dynamicdata)  [unwired: 3 in]
                n223 = call "Convert to Dynamic Data121"("Array"=w341) -> ("Dynamic Data Type"=w340:dynamicdata)  [unwired: 3 in]
                n224 = call "Convert to Dynamic Data135"("Array"=w331) -> ("Dynamic Data Type"=w330:dynamicdata)  [unwired: 3 in]
                n225 = call "Convert to Dynamic Data134"("Array"=w333) -> ("Dynamic Data Type"=w332:dynamicdata)  [unwired: 3 in]
                n226 = call "Convert to Dynamic Data123"("Array"=w345) -> ("Dynamic Data Type"=w344:dynamicdata)  [unwired: 3 in]
                n227 = call "Convert to Dynamic Data127"("Array"=w353) -> ("Dynamic Data Type"=w352:dynamicdata)  [unwired: 3 in]
                n228 = call "Convert to Dynamic Data133"("Array"=w335) -> ("Dynamic Data Type"=w334:dynamicdata)  [unwired: 3 in]
                n229 = call "Convert to Dynamic Data128"("Array"=w355) -> ("Dynamic Data Type"=w354:dynamicdata)  [unwired: 3 in]
                n230 = call "Convert to Dynamic Data124"("Array"=w347) -> ("Dynamic Data Type"=w346:dynamicdata)  [unwired: 3 in]
                n231 = call "Convert to Dynamic Data122"("Array"=w343) -> ("Dynamic Data Type"=w342:dynamicdata)  [unwired: 3 in]
                n232 = call "Convert to Dynamic Data132"("Array"=w337) -> ("Dynamic Data Type"=w336:dynamicdata)  [unwired: 3 in]
                n233 = call "Convert to Dynamic Data136"("Array"=w329) -> ("Dynamic Data Type"=w328:dynamicdata)  [unwired: 3 in]
                n234 = Merge Signals(w359, w361, w354, w352, w350, w348, w346, w344, w342, w340, w338, w336, w334, w332, w330, w328) -> (w357:dynamicdata)
              }
              frame 1, Default {
                n235 = Decimate 1D Array(w362) -> (w364:i32[])
                n236 = call "Convert to Dynamic Data3"("Array"=w364) -> ("Dynamic Data Type"=w365:dynamicdata)  [unwired: 3 in]
                n237 = Merge Signals(w365) -> (w363:dynamicdata)
              }
            }
            "Waveform Graph" <- w41
          }
        }
        frame True {
          n238 = call "Display Message to User2"() -> ()  [unwired: 10 in, 2 out]
        }
      }
      n239 = flat-sequence {
        tunnel: w20 -> [w470]
        frame #0 {
          # "HRDLStop"
          # "HRDLCloseUnit"
          n240 = dll-call lib="picohrdl.dll" fn="HRDLStop"("handle"=w470) -> ("handle"=w471:i16)  [unwired: 4 in, 2 out]
          n241 = dll-call lib="PicoHRDL.dll" fn="HRDLCloseUnit"("handle"=w471) -> ()  [unwired: 5 in, 2 out]
        }
        frame #1 {
          n242 = local write "stop"(FALSE ("stop")) -> ()
        }
      }
    }
  }
